vi "Server.vi"(8 "error in (no error)":errorcluster, 10 "Queue Name":string) -> (0 "error out":errorcluster)   [LabVIEW 2011]
doc: "This is the server in the QDMH Client - Server example. This demonstration illustrates one way to take the existing QDMH and extend funtionality. Multiple clients can \"connect\" to the server. Examine the block diagram to see how the server keeps track of which client has made a connection. This is an illustration of leveraging the flexiblitiy of named queues.\n\nAAL 9/09"
uses:
  Shared/QDMH Poly VIs/QDMH POLY Enqueue String.vi
  Shared/QDMH Poly VIs/QDMH POLY Enqueue Cluster.vi
panel:
  in  "Simulated Data":dbl
  in  "Get Data":bool
  out "Message Display":string
  in  "Cancel":bool
  in  "OK":bool
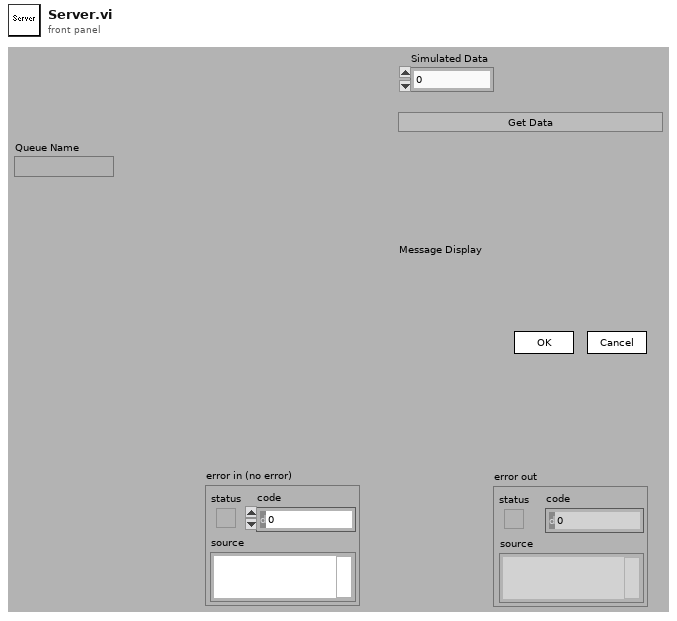
[diagram p1: front panel]
types:
  T1 = cluster{"Operator Name":string, "Current VI's Path":path, "Current VI's  Directory":path, "Queue Names":string[], "# VIs Launched":i32, "Simulated Data":dbl}
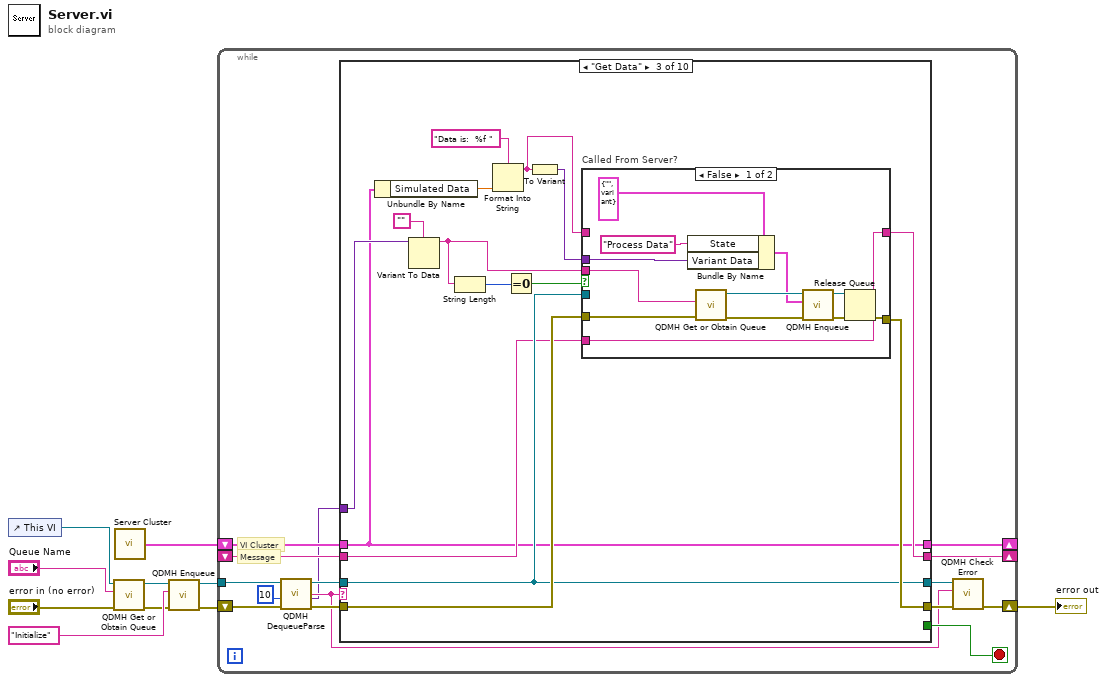
[diagram p0: block diagram]
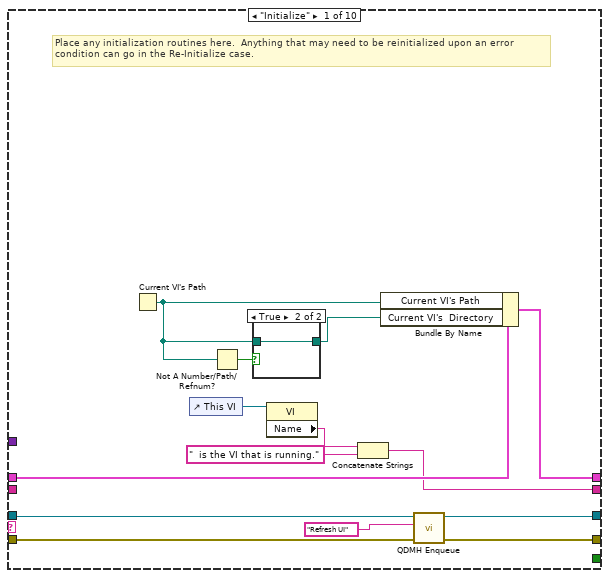
[diagram p2: hidden frame]
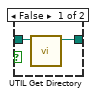
[diagram p3: hidden frame]
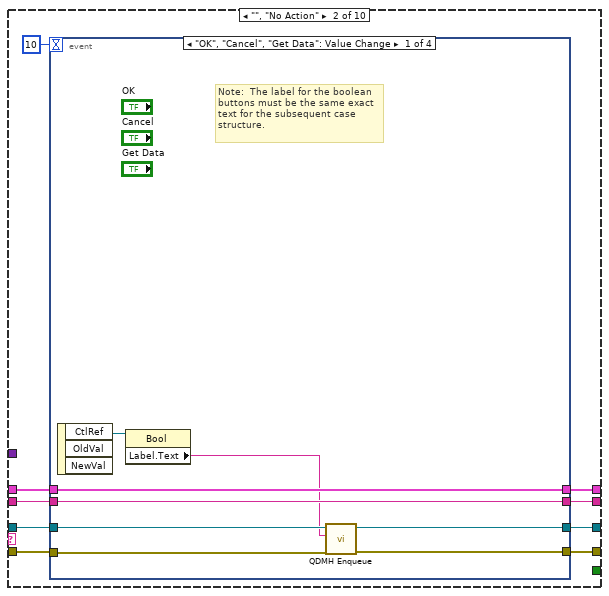
[diagram p4: hidden frame]
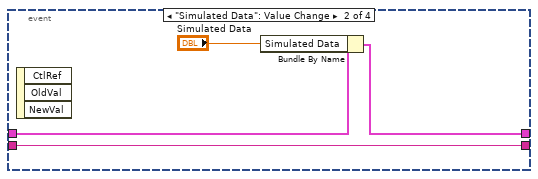
[diagram p5: hidden frame]
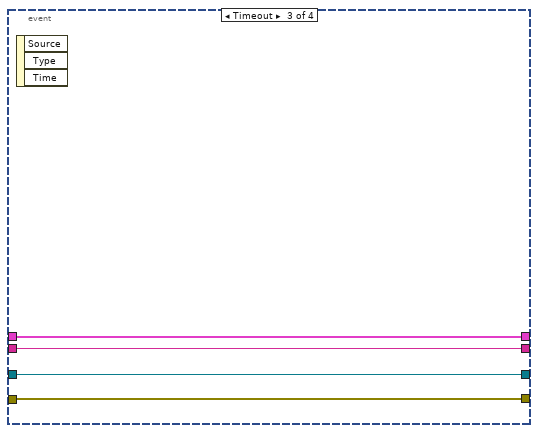
[diagram p6: hidden frame]
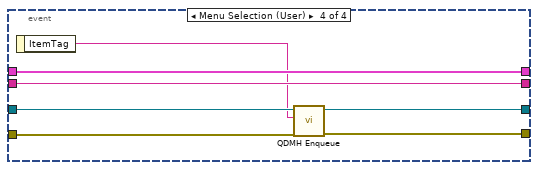
[diagram p7: hidden frame]
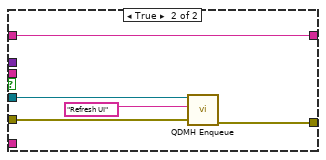
[diagram p8: hidden frame]
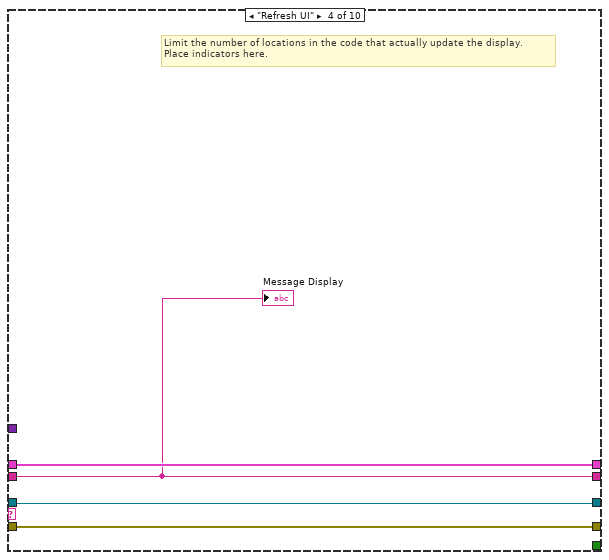
[diagram p9: hidden frame]
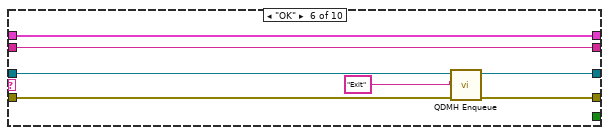
[diagram p11: hidden frame]
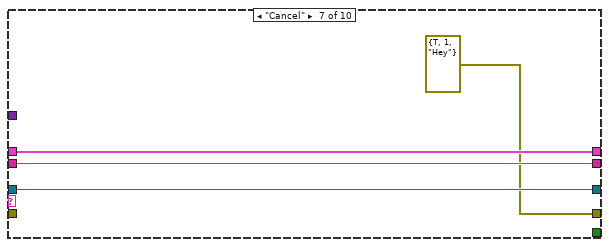
[diagram p12: hidden frame]
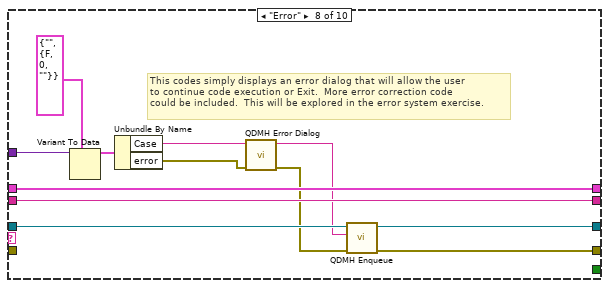
[diagram p13: hidden frame]
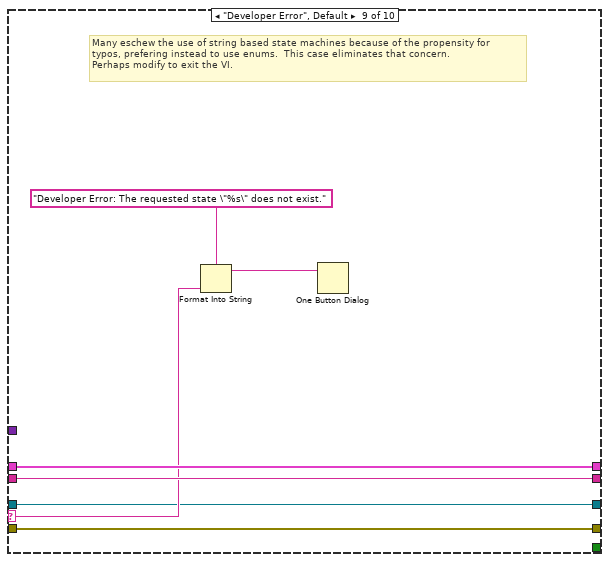
[diagram p14: hidden frame]
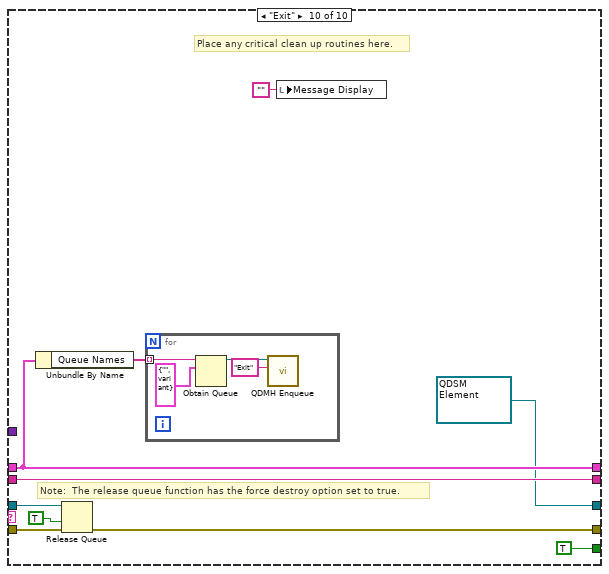
[diagram p15: hidden frame]
diagram:
  n1 = control-ref of="This VI"() -> (w1:refnum<vi>)
  n2 = call "QDMH Get or Obtain Queue.vi"("error in (no error)"="error in (no error)", "Queue Name"="Queue Name", "VI Refnum"=w1) -> ("error out"=w4:errorcluster, "queue out"=w5:refnum<queue>)  [unwired: 7 out]
  n3 = call "Server Cluster.vi"() -> ("Cluster"=w10:T1)
  n4 = call-poly "QDMH Enqueue.vi"("error in (no error)"=w4, "State"="Initialize" ("element"), "queue"=w5) -> ("error out"=w2:errorcluster, "queue out"=w3:refnum<queue>)  [unwired: 7 out]
  n5 = while {
    tunnel: w3 -> [w20]
    shift-left: w10 -> [w21]
    shift-right: [w22] -> _
    shift-left: _ -> [w23]
    shift-right: [w24] -> _
    shift-right: [w14] -> w8
    shift-left: w2 -> [w16]
    stop <- w25 stop-if-true
    # "VI Cluster"
    # "Message"
    n6 = call "QDMH DequeueParse.vi"("error in (no error)"=w16, "Timeout"=10 ("ms timeout (-1)"), "queue"=w20) -> ("error out"=w17:errorcluster, "Variant Data"=w11:variant, "State"=w12:string, "queue out"=w18:refnum<queue>)  [unwired: 5 out]
    n7 = case shown="\"Get Data\"" w12 {
      selector: w12 -> [_ _ _ _ _ _ _ _ w141 _]
      tunnel: w18 -> [w35 w51 w79 w108 w111 w121 w123 w135 w138 w151]
      tunnel: [_ _ _ _ _ _ _ _ _ TRUE] -> w25
      tunnel: [w33 w44 w77 w109 w114 w120 w125 w137 w144 w153] -> w24
      tunnel: w23 -> [_ w45 w78 w109 w114 w120 w125 w137 w144 w153]
      tunnel: [w38 w46 w76 w110 w113 w119 w124 w136 w143 w148] -> w22
      tunnel: w21 -> [w39 w47 w76 w110 w113 w119 w124 w136 w143 w148]
      tunnel: w17 -> [w37 w50 w81 w107 w112 w118 _ _ w140 w150]
      tunnel: [w36 w49 w80 w107 w112 w117 errorcluster {"status"=TRUE, "code"=1, "source"="Hey"} ("error out") w134 w140 w145] -> w15
      tunnel: [w28 w43 w79 w108 w111 w115 w123 w133 w138 refnum<queue> refnum ("queue out")] -> w13
      tunnel: w11 -> [_ _ w82 _ _ _ _ w131 _ _]
      frame "Initialize" {
        # "Place any initialization routines here.  Anything that may need to be reinitialized upon an error\ncondition can go in the Re-Initialize case."
        n8 = Current VI's Path() -> (path=w26:path)
        n9 = control-ref of="This VI"() -> (w32:refnum<vi>)
        n10 = Not A Number/Path/Refnum?(number/path/refnum=w26) -> (NaN/Path/Refnum?=w27:bool)
        n11 = case shown="True" w27 {
          tunnel: w26 -> [w41 w42]
          tunnel: [w40 w42] -> w30
          frame False {
            n12 = call "UTIL Get Directory.vi"("Path In"=w41) -> ("Directory Out"=w40:path)  [unwired: 1 in, 9 out]
          }
          frame True {
          }
        }
        n13 = property class="VI"(reference=w32) -> ("Name"=w31:string)  [unwired: 1 in, 2 out]
        n14 = Concatenate Strings(w31, "  is the VI that is running." ("string")) -> (w33:string)
        n15 = Bundle By Name(cluster=w39, "Current VI's Path"=w26, "Current VI's  Directory"=w30) -> (w38:T1)
        n16 = call-poly "QDMH Enqueue.vi"("error in (no error)"=w37, "State"="Refresh UI" ("New State"), "queue"=w35) -> ("error out"=w36:errorcluster, "queue out"=w28:refnum<queue>)  [unwired: 7 out]
      }
      frame "", "No Action" {
        n17 = event shown="[0] \"OK\", \"Cancel\", \"Get Data\": Value Change" {
          selector: _ -> [_ _ _ _]
          dyn-events: _ -> [_ _ _ _]
          timeout: 10 -> [_ _ _ _]
          tunnel: w51 -> [w58 _ w64 w74]
          tunnel: [w57 _ w67 w72] -> w49
          tunnel: w50 -> [w56 _ w67 w73]
          tunnel: w47 -> [w55 w61 w66 w71]
          tunnel: [w55 w60 w66 w71] -> w46
          tunnel: w45 -> [w54 w63 w65 w70]
          tunnel: [w54 w63 w65 w70] -> w44
          tunnel: [w52 _ w64 w68] -> w43
          event "OK", "Cancel", "Get Data": Value Change {
            # "Note:  The label for the boolean buttons must be the same exact text for the subsequent case structure."
            n18 = event-data() -> ("CtlRef"=w59:refnum<vi>)  [unwired: 3 out]
            n19 = property class="Bool"(reference=w59) -> ("Label.Text"=w53:string)  [unwired: 1 in, 2 out]
            n20 = call-poly "QDMH Enqueue.vi"("error in (no error)"=w56, "State"=w53, "queue"=w58) -> ("error out"=w57:errorcluster, "queue out"=w52:refnum<queue>)  [unwired: 7 out]
          }
          event "Simulated Data": Value Change {
            n21 = event-data() -> ()  [unwired: 4 out]
            n22 = Bundle By Name(cluster=w61, "Simulated Data"="Simulated Data") -> (w60:T1)
          }
          event Timeout {
            n23 = event-data() -> ()  [unwired: 4 out]
          }
          event Menu Selection (User) {
            n24 = event-data() -> ("ItemTag"=w69:string)  [unwired: 1 out]
            n25 = call-poly "QDMH Enqueue.vi"("error in (no error)"=w73, "State"=w69, "queue"=w74) -> ("error out"=w72:errorcluster, "queue out"=w68:refnum<queue>)  [unwired: 7 out]
          }
        }
      }
      frame "Get Data" {
        n26 = Unbundle By Name(w76) -> ("Simulated Data"=w75:dbl)
        n27 = Variant To Data(type="", Variant=w82) -> (data=w86:string)  [unwired: 1 in, 1 out]
        n28 = String Length(string=w86) -> (length=w85:i32)
        n29 = Format Into String(format string="Data is:  %f ", w75) -> (resulting string=w89:string)  [unwired: 2 in, 1 out]
        n30 = Equal To 0?(x=w85) -> (x = 0?=w84:bool)
        n31 = To Variant(anything=w89) -> (Variant=w88:variant)
        n32 = case "Called From Server?" shown="False" w84 {
          tunnel: w78 -> [w101 _]
          tunnel: w88 -> [w96 _]
          tunnel: [w101 w103] -> w77
          tunnel: w79 -> [_ w106]
          tunnel: w81 -> [w100 w105]
          tunnel: [w92 w104] -> w80
          tunnel: w86 -> [w94 _]
          tunnel: w89 -> [_ w103]
          frame False {
            n33 = Bundle By Name(cluster=cluster{"State":string, "Variant Data":variant} {"State"="", "Variant Data"=variant} ("QDSM Element"), "State"="Process Data", "Variant Data"=w96) -> (w95:cluster{"State":string, "Variant Data":variant})
            n34 = call "QDMH Get or Obtain Queue.vi"("error in (no error)"=w100, "Queue Name"=w94) -> ("error out"=w99:errorcluster, "queue out"=w98:refnum<queue>)  [unwired: 1 in, 7 out]
            n35 = call-poly "QDMH Enqueue.vi"("error in (no error)"=w99, "QDSM Element"=w95, "queue"=w98) -> ("error out"=w91:errorcluster, "queue out"=w90:refnum<queue>)  [unwired: 7 out]
            n36 = Release Queue(queue=w90, error in (no error)=w91) -> (error out=w92:errorcluster)  [unwired: 3 out]
          }
          frame True {
            n37 = call-poly "QDMH Enqueue.vi"("error in (no error)"=w105, "State"="Refresh UI" ("New State"), "queue"=w106) -> ("error out"=w104:errorcluster)  [unwired: 8 out]
          }
        }
      }
      frame "Refresh UI" {
        # "Limit the number of locations in the code that actually update the display.\nPlace indicators here."
        "Message Display" <- w109
      }
      frame "<duplicate me for new states >" {
      }
      frame "OK" {
        n38 = call-poly "QDMH Enqueue.vi"("error in (no error)"=w118, "State"="Exit" ("New State"), "queue"=w121) -> ("error out"=w117:errorcluster, "queue out"=w115:refnum<queue>)  [unwired: 7 out]
      }
      frame "Cancel" {
      }
      frame "Error" {
        # "This codes simply displays an error dialog that will allow the user\nto continue code execution or Exit.  More error correction code\ncould be included.  This will be explored in the error system exercise."
        n39 = Variant To Data(type=cluster{"Case":string, "error":errorcluster} {"Case"="", "error"={"status"=FALSE, "code"=0, "source"=""}} ("QDSM Element"), Variant=w131) -> (data=w130:cluster{"Case":string, "error":errorcluster})  [unwired: 1 in, 1 out]
        n40 = Unbundle By Name(w130) -> ("Case"=w129:string, "error"=w128:errorcluster)
        n41 = call "QDMH Error Dialog.vi"("error"=w128, "Case Error Occured"=w129) -> ("error out (no error)"=w126:errorcluster, "Case to Execute"=w127:string)  [unwired: 8 out]
        n42 = call-poly "QDMH Enqueue.vi"("error in (no error)"=w126, "State"=w127, "queue"=w135) -> ("error out"=w134:errorcluster, "queue out"=w133:refnum<queue>)  [unwired: 7 out]
      }
      frame "Developer Error", Default {
        # "Many eschew the use of string based state machines because of the propensity for\ntypos, prefering instead to use enums.  This case eliminates that concern.\nPerhaps modify to exit the VI."
        n43 = Format Into String(format string="Developer Error: The requested state \"%s\" does not exist." ("message"), w141) -> (resulting string=w139:string)  [unwired: 2 in, 1 out]
        n44 = One Button Dialog(message=w139) -> ()  [unwired: 2 out]
      }
      frame "Exit" {
        # "Note:  The release queue function has the force destroy option set to true."
        # "Place any critical clean up routines here."
        n45 = Unbundle By Name(w148) -> ("Queue Names"=w146:string[])
        n46 = Release Queue(queue=w151, force destroy? (F)=TRUE, error in (no error)=w150) -> (error out=w145:errorcluster)  [unwired: 2 out]
        n47 = for {
          tunnel: w146 -> [w158] mode=indexing
          n48 = Obtain Queue(name (unnamed)=w158, element data type=cluster{"State":string, "Variant Data":variant} {"State"="", "Variant Data"=variant} ("QDSM Element")) -> (queue out=w157:refnum<queue>)  [unwired: 3 in, 2 out]
          n49 = call-poly "QDMH Enqueue.vi"("State"="Exit" ("element"), "queue"=w157) -> ()  [unwired: 1 in, 9 out]
        }
        n50 = local write "Message Display"("") -> ()
      }
    }
    n51 = call "QDMH Check Error.vi"("error in (no error)"=w15, "Case"=w12, "queue"=w13) -> ("error out"=w14:errorcluster)  [unwired: 1 in, 7 out]
  }
  "error out" <- w8
